vi "Automatic_Parking_System_VI.vi"() -> ()   [LabVIEW 2024]
panel:
  out "Data":string
  out "Time":string
  in  "Switcher":bool
  out "Slot  data":string
  out "Slot 1 Full":bool
  out "Slot 1 empty":bool
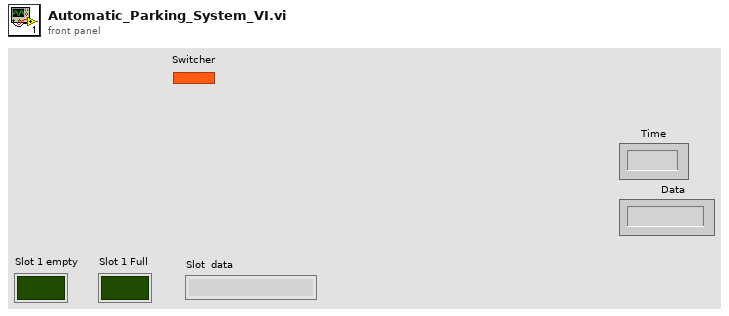
[diagram p1: front panel]
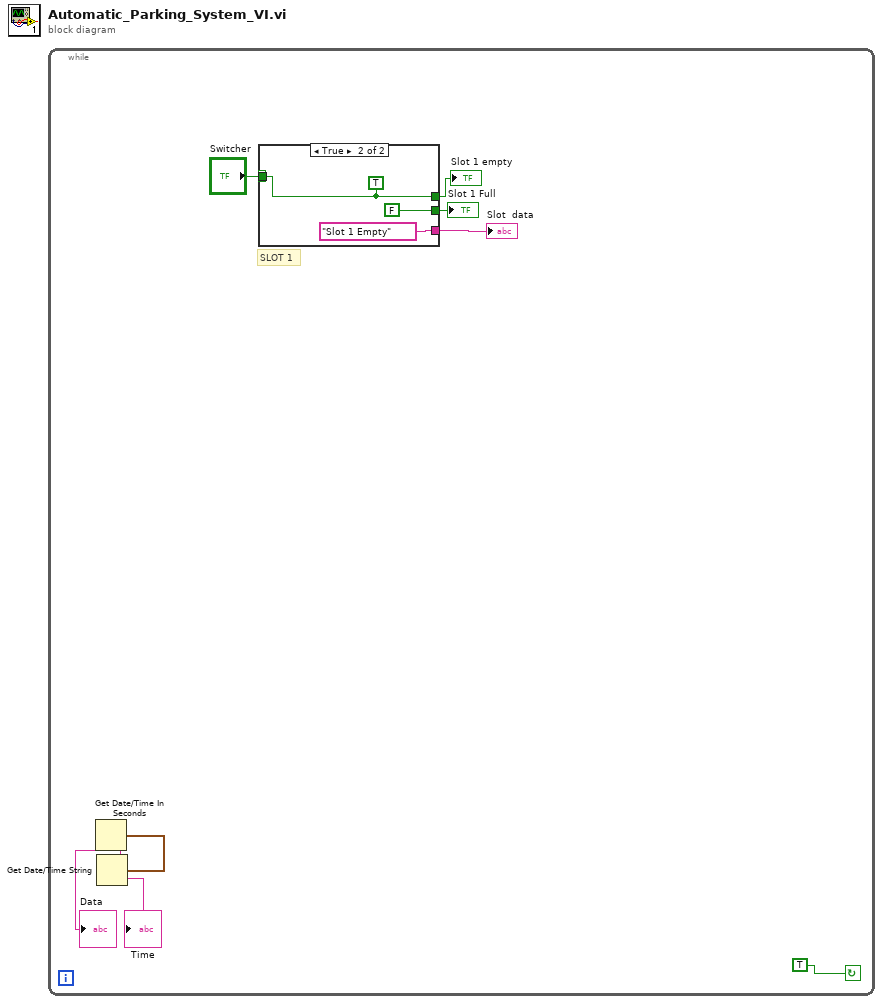
[diagram p0: block diagram]
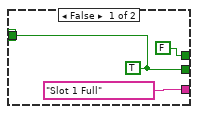
[diagram p2: hidden frame]
diagram:
  n1 = while {
    stop <- TRUE continue-if-true
    # "SLOT 1"
    n2 = Get Date/Time In Seconds() -> (seconds since 1Jan1904=w2:timestamp)
    n3 = Get Date/Time String(seconds (now)=w2) -> (date string=→"Data":string, time string=→"Time":string)  [unwired: 2 in]
    n4 = case shown="True" "Switcher" {
      selector: "Switcher" -> [w11 w15]
      tunnel: ["Slot 1 Full" "Slot 1 Empty"] -> w7
      tunnel: [w11 w13] -> _
      tunnel: [w9 w15] -> _
      tunnel: [FALSE w13] -> w5
      tunnel: [w9 FALSE] -> w4
      frame False {
        w9 = TRUE
      }
      frame True {
        w13 = TRUE
      }
    }
    "Slot  data" <- w7
    "Slot 1 Full" <- w4
    "Slot 1 empty" <- w5
  }
